vi "SetParam.vi"(8 "error in (no error)":errorcluster caption="entrée d'erreur (pas d'erreur)", 10 "ShuffleSplit":T1={"n_splits"=10, "test_size"="None", "train_size"="None", "random_state"=-1} {"random_state" min=-1}, 11 "ShuffleSplit.lvclass":refnum<class "ShuffleSplit.lvclass">) -> (0 "error out":errorcluster caption="sortie d'erreur", 3 "ShuffleSplit.lvclass":refnum<class "ShuffleSplit.lvclass">)   [LabVIEW 2020, in "ShuffleSplit.lvclass"]
doc: "Set Parameters"
uses:
  ShuffleSplit.lvclass
  ShuffleSplit.lvclass/ShuffleSplit.ctl
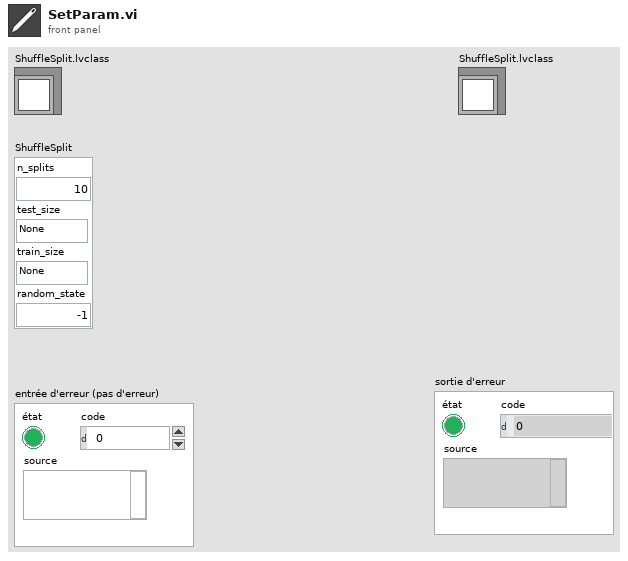
[diagram p1: front panel]
types:
  T1 = cluster{"n_splits":i32, "test_size":string, "train_size":string, "random_state":i32}
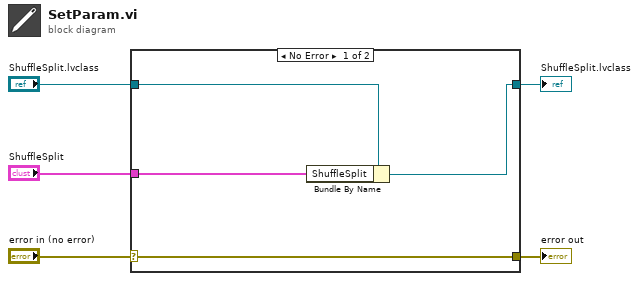
[diagram p0: block diagram]
diagram:
  n1 = case shown="No Error" "error in (no error)" {
    selector: "error in (no error)" -> [w9 w10]
    tunnel: [w9 w10] -> w4
    tunnel: [w7 w11] -> w2
    tunnel: "ShuffleSplit.lvclass" -> [w8 w11]
    tunnel: "ShuffleSplit" -> [w6 _]
    frame No Error {
      n2 = Bundle By Name(cluster=w8, "ShuffleSplit"=w6) -> (w7:refnum<class "ShuffleSplit.lvclass">)
    }
    frame Error {
    }
  }
  "error out" <- w4
  "ShuffleSplit.lvclass" <- w2
